vi "Write Coordinates.CAD Cluster.vi"(8 "error in (no error)":errorcluster, 10 "Coordinates.CAD Cluster":T1(array[cluster]), 11 "CAD Dispense in":refnum<class "CAD Dispense.lvclass">) -> (0 "error out":errorcluster, 3 "CAD Dispense out":refnum<class "CAD Dispense.lvclass">)   [LabVIEW 2020, in "CAD Dispense.lvclass"]
uses:
  CAD Dispense.lvclass
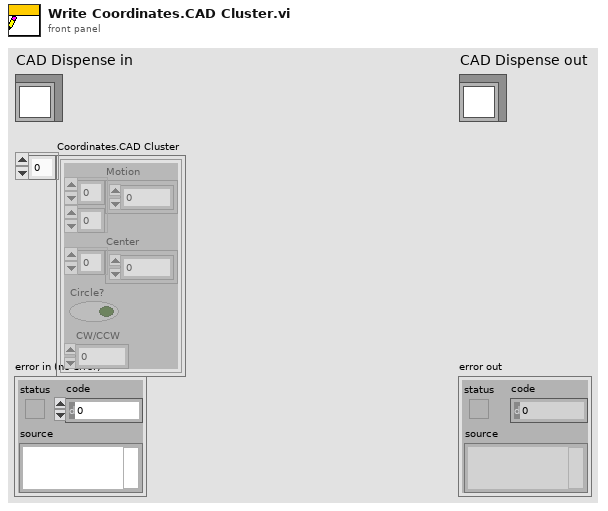
[diagram p1: front panel]
types:
  T1 = cluster{"Motion":dbl[][], "Center":dbl[], "Circle?":bool, "CW/CCW":dbl}[]
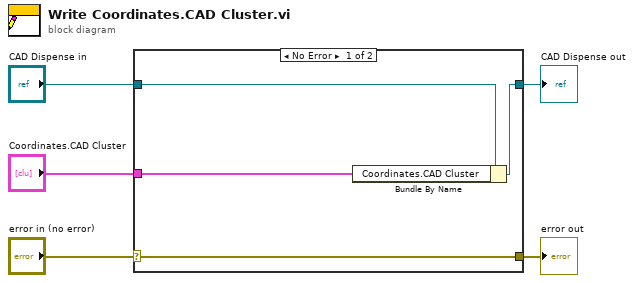
[diagram p0: block diagram]
diagram:
  n1 = case shown="No Error" "error in (no error)" {
    selector: "error in (no error)" -> [w9 w10]
    tunnel: [w9 w10] -> w4
    tunnel: [w7 w11] -> w2
    tunnel: "CAD Dispense in" -> [w8 w11]
    tunnel: "Coordinates.CAD Cluster" -> [w6 _]
    frame No Error {
      n2 = Bundle By Name(cluster=w8, "Coordinates.CAD Cluster"=w6) -> (w7:refnum<class "CAD Dispense.lvclass">)
    }
    frame Error {
    }
  }
  "error out" <- w4
  "CAD Dispense out" <- w2
